vi "Calculator by Eason023.vi"() -> ()   [LabVIEW 2021]
uses:
  <vilib>/regexp/Match Regular Expression.xnode
  <vilib>/gmath/NI_Gmath.lvlib
panel:
  out "Display":string
  in  "C Button":bool
  in  "Stop button":bool
  in  "?":bool
  out "?":bool
  out "?":bool
  out "?":bool
  out "?":bool
  out "?":bool
  out "?":bool
  out "?":bool
  out "?":bool
  out "?":bool
  out "?":bool
  out "?":bool
  out "?":bool
  out "?":bool
  out "?":bool
  out "?":bool
  out "?":bool
  out "?":bool
  out "?":bool
  out "?":bool
  out "?":bool
  out "?":bool
  out "?":bool
  out "?":bool
  out "?":bool
  out "?":bool
  out "?":bool
  out "?":bool
  out "?":bool
  out "?":bool
  out "?":bool
  out "?":bool
  out "?":bool
  out "?":bool
  out "?":bool
  out "?":bool
  out "?":bool
  out "?":bool
  out "?":bool
  out "?":bool
  out "?":bool
  out "?":bool
  out "?":bool
  out "?":bool
  out "?":bool
  out "?":bool
  out "?":bool
  out "?":bool
  out "?":bool
  out "?":bool
  out "?":bool
  out "?":bool
  out "?":bool
  out "?":bool
  out "?":bool
  out "?":bool
  out "?":bool
  out "?":bool
  out "?":bool
  out "?":bool
  out "?":bool
  out "?":bool
  out "?":bool
  out "?":bool
  out "?":bool
  out "?":bool
  out "?":bool
  out "?":bool
  out "?":bool
  out "?":bool
  out "?":bool
  out "?":bool
  out "Elapsed time (s)":u32
  out "Current Time":timestamp
  in  "Load From B Button":bool
  in  "Load From A Button":bool
  in  "Save Button":bool caption="2 Button"
  out "Memory B :":string
  out "Memory A :":string
  in  "1/x Button":bool caption="2 Button"
  in  "≡ Button":bool caption="2 Button"
  in  "+/- Button":bool caption="2 Button"
  in  "CE Button":bool
  in  "\"=\" Button":bool
  out "Syntax Error\nWarning":bool
  in  "Backspace Button":bool
  in  "\")\" Button":bool
  in  "\"(\" Button":bool
  in  "'+' Button":bool caption="2 Button"
  in  "'-' Button":bool caption="2 Button"
  in  "'*' Button":bool caption="2 Button"
  in  "'/' Button":bool caption="2 Button"
  in  "'.' Button":bool caption="2 Button"
  in  "0 Button":bool caption="2 Button"
  in  "8 Button":bool caption="2 Button"
  in  "6 Button":bool caption="2 Button"
  in  "4 Button":bool caption="2 Button"
  in  "9 Button":bool caption="2 Button"
  in  "7 Button":bool caption="2 Button"
  in  "5 Button":bool caption="2 Button"
  in  "3 Button":bool caption="2 Button"
  in  "2 Button":bool
  in  "1 Button":bool
  out "?":bool
  # "七段顯示器 最多10位 (整數與小數各5位) 僅顯示結果 (\"=\"後的數) 超出部分不顯示"
  # "Display mod:\nDetailed----Simple"
  # "Calculator\n          by 113550153"
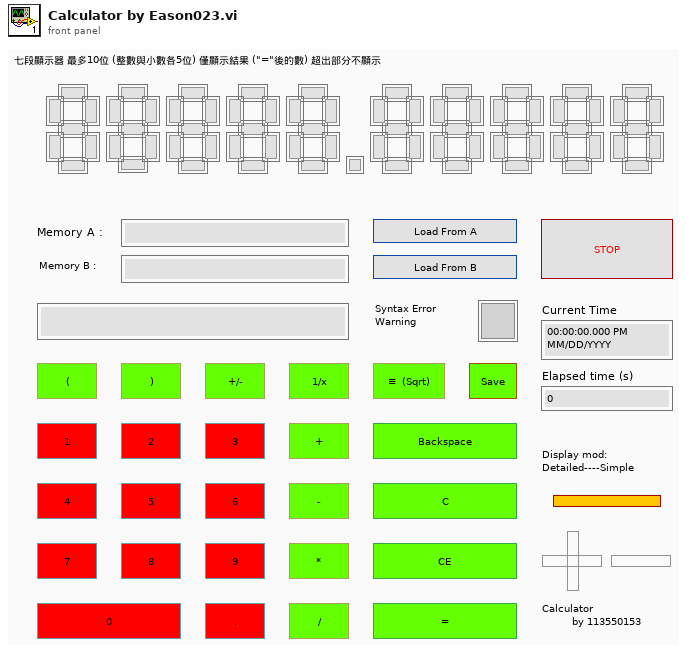
[diagram p1: front panel]
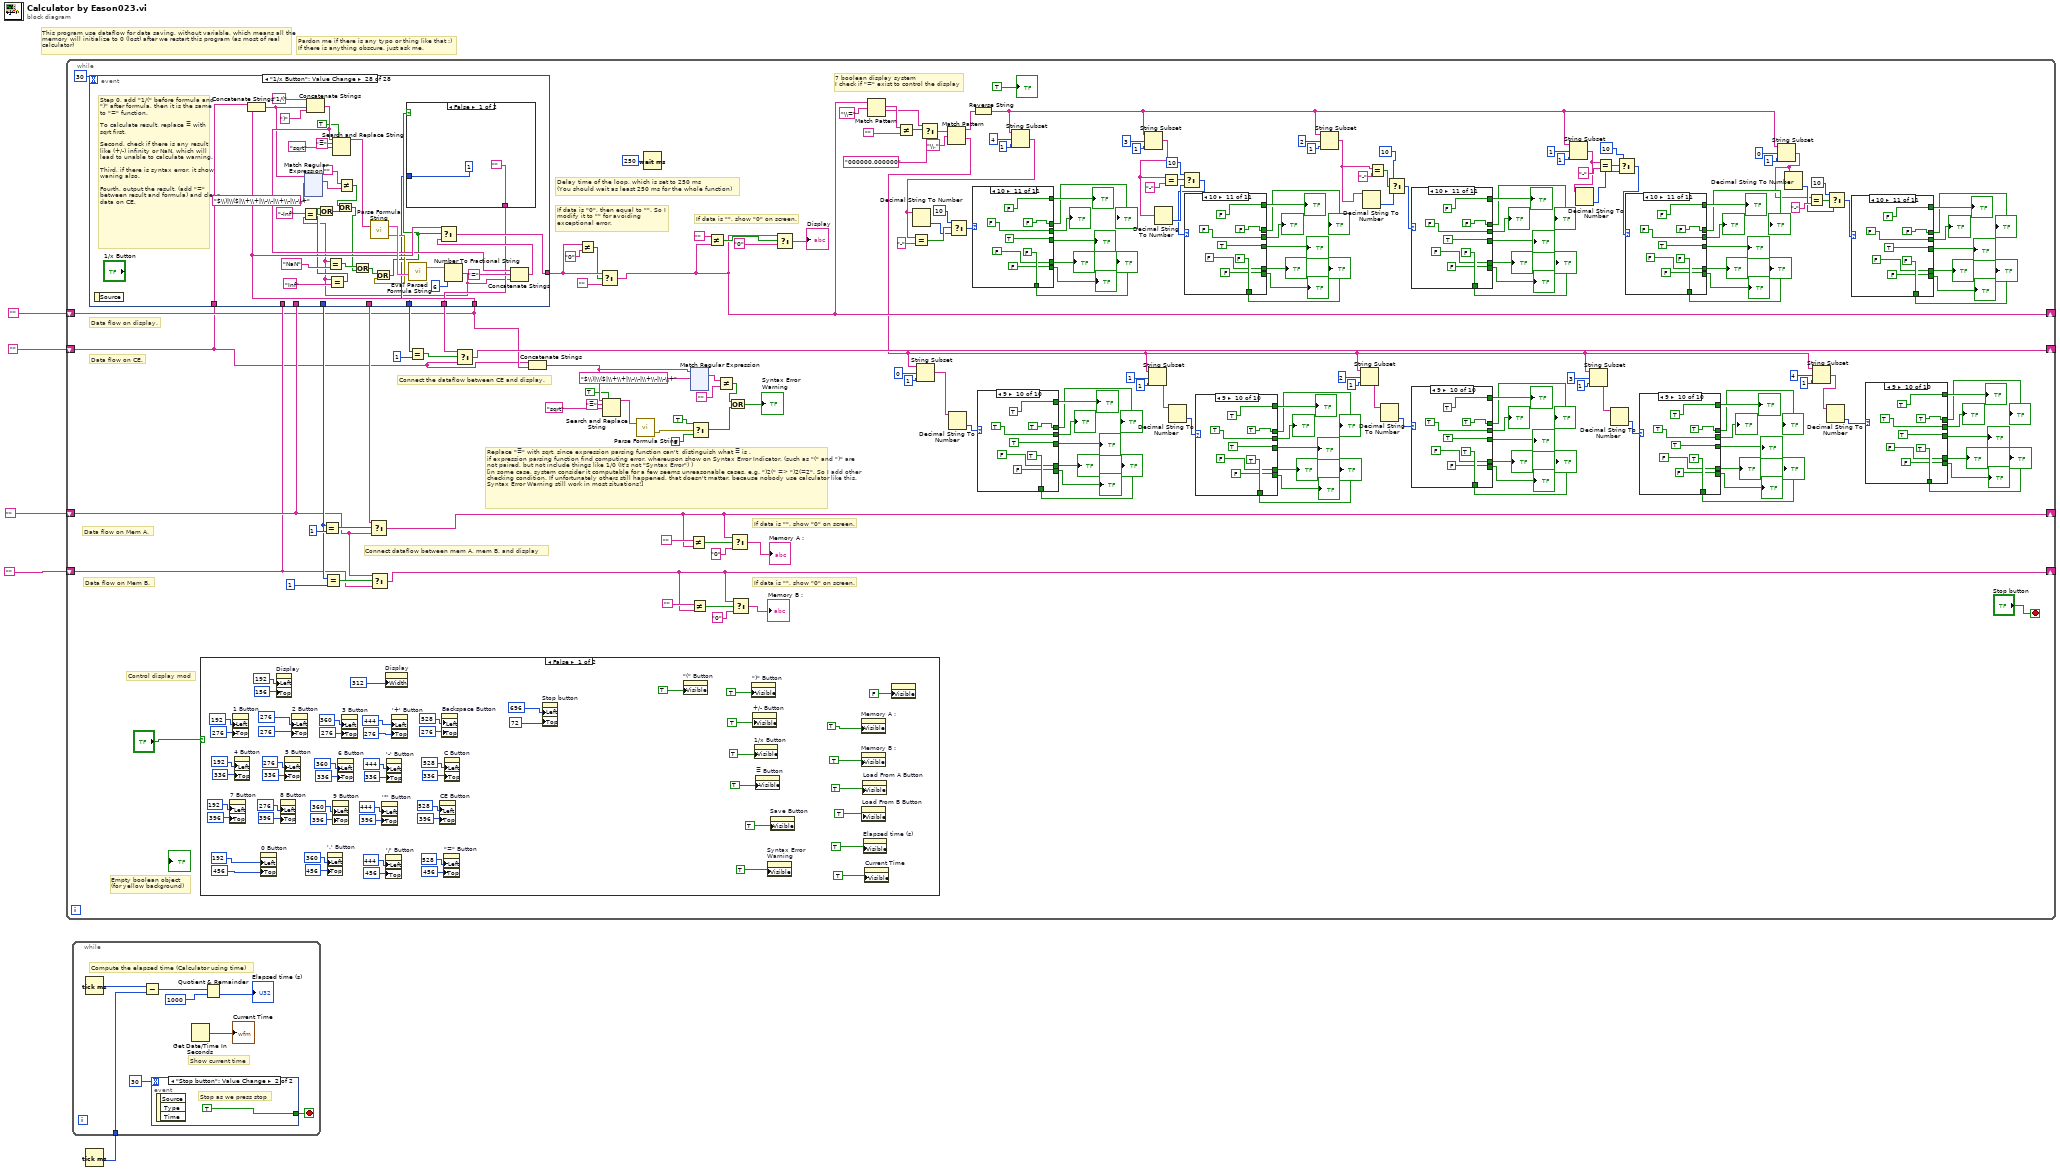
[diagram p0: block diagram]
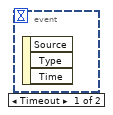
[diagram p2: hidden frame]
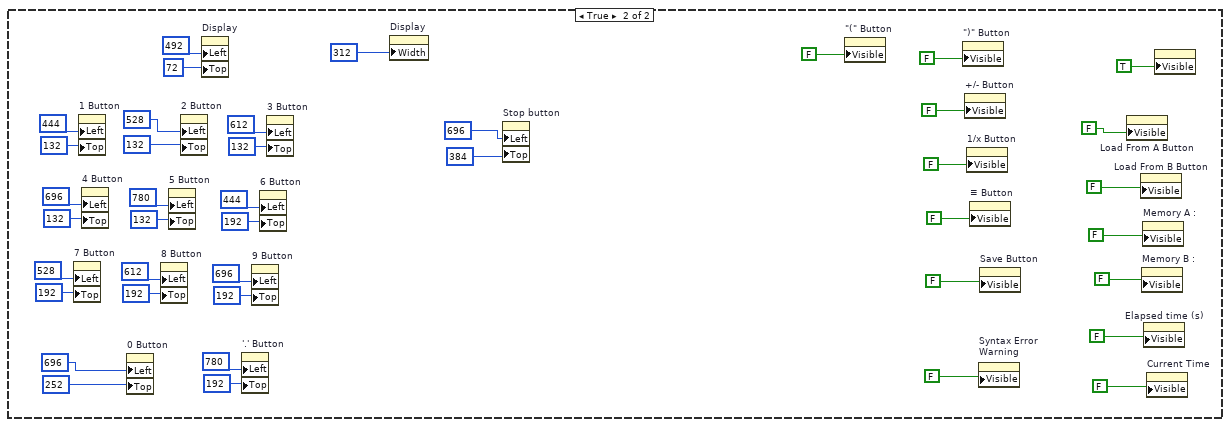
[diagram p3: hidden frame]
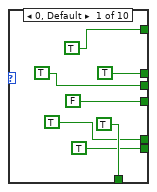
[diagram p4: hidden frame]
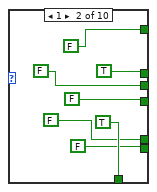
[diagram p5: hidden frame]
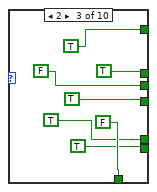
[diagram p6: hidden frame]
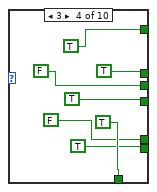
[diagram p7: hidden frame]
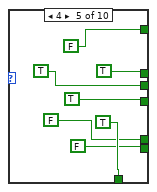
[diagram p8: hidden frame]
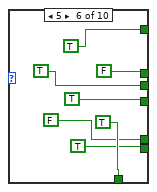
[diagram p9: hidden frame]
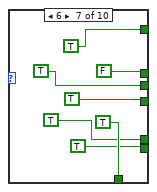
[diagram p10: hidden frame]
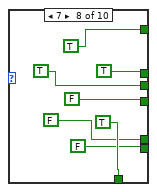
[diagram p11: hidden frame]
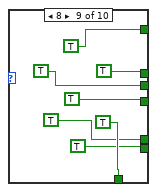
[diagram p12: hidden frame]
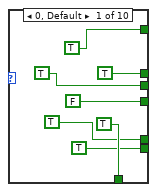
[diagram p13: hidden frame]
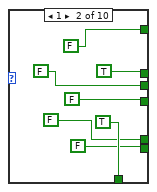
[diagram p14: hidden frame]
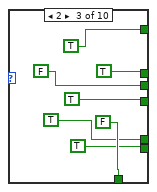
[diagram p15: hidden frame]
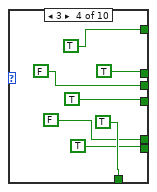
[diagram p16: hidden frame]
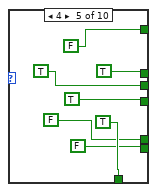
[diagram p17: hidden frame]
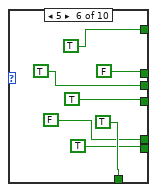
[diagram p18: hidden frame]
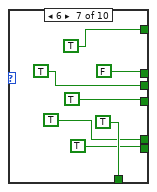
[diagram p19: hidden frame]
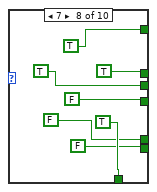
[diagram p20: hidden frame]
diagram:
  # "Pardon me if there is any typo or thing like that :)\nIf there is anything obscure, just ask me."
  # "This program use dataflow for data saving, without variable, which means all the memory will initialize to 0 (lost) after we restart this program (as most of real calculator)"
  n1 = while {
    shift-right: [w156] -> _
    shift-left: "" -> [w161]
    shift-right: [w186] -> _
    shift-left: "" -> [w160]
    shift-right: [w171] -> _
    shift-left: "" -> [w169]
    shift-right: [w173] -> _
    shift-left: "" -> [w168]
    stop <- "Stop button" stop-if-true
    # "Empty boolean object\n(for yellow background)"
    # "Control display mod"
    # "7 boolean display system\nI check if \"=\" exist to control the display"
    # "If data is \"\", show \"0\" on screen."
    # "If data is \"\", show \"0\" on screen."
    # "Connect dataflow between mem A, mem B, and display"
    # "Delay time of the loop, which is set to 250 ms\n(You should wait as least 250 ms for the whole function)"
    # "Connect the dataflow between CE and display."
    # "Replace \"≡\" with sqrt, since expression parsing function can't  distinguish what ≡ is .\nif expression parsing function find computing error, whereupon show on Syntax Error Indicator. (such as \"(\" and \")\" are not paired, but not include things like 1/0 (It's not \"Syntax Error\") )\n[in some case, system consider it computable for a few seems unreasonable cases, e.g. \")2(\" => \")2(=2\". So I add other checking condition. If unfortunately others still happened, that doesn't matter, because nobody use calculator like this. Syntax Error Warning still work in most situations!]"
    # "Data flow on Mem B."
    # "Data flow on Mem A."
    # "Data flow on CE."
    # "Data flow on display."
    # "If data is \"\", show \"0\" on screen."
    # "If data is \"0\", then equal to \"\". So I modify it to \"\" for avoiding\nexceptional error."
    n2 = event shown="[27] \"1/x Button\": Value Change" {
      selector: _ -> [_ _ _ _ _ _ _ _ _ _ _ _ _ _ _ _ _ _ _ _ _ _ _ _ _ _ _ _]
      dyn-events: _ -> [_ _ _ _ _ _ _ _ _ _ _ _ _ _ _ _ _ _ _ _ _ _ _ _ _ _ _ _]
      timeout: 30 -> [_ _ _ _ _ _ _ _ _ _ _ _ _ _ _ _ _ _ _ _ _ _ _ _ _ _ _ _]
      tunnel: w161 -> [w1150 w1152 w1155 w1158 w1161 w1164 w1167 w1170 w1173 w1176 w1179 w1186 w1203 w1206 w1209 w1212 w1215 w1218 w1232 w1354 w1357 w1370 w1372 w1387 _ _ w2040 w2193]
      tunnel: [w1150 w1151 w1154 w1157 w1160 w1163 w1166 w1169 w1172 w1175 w1182 w1196 w1204 w1207 w1210 w1213 w1216 w1219 w1234 "" w1358 w1369 w1372 w1418 w2012 w2013 w2042 w2195] -> w194
      tunnel: [_ _ _ _ _ _ _ _ _ _ _ _ _ _ _ _ _ _ _ i8 1 w1359 _ _ _ _ _ w2029 w2179] -> w189
      tunnel: [_ _ _ _ _ _ _ _ _ _ _ _ _ _ _ _ _ _ _ w1354 w1360 _ _ _ _ _ w2028 w2178] -> w187
      tunnel: [_ _ _ _ _ _ _ _ _ _ _ _ _ _ _ _ _ _ _ _ _ _ i8 1 _ _ _ _ _] -> w181
      tunnel: [_ _ _ _ _ _ _ _ _ _ _ _ _ _ _ _ _ _ _ _ _ _ w1372 _ _ _ _ _] -> w183
      tunnel: w169 -> [_ _ _ _ _ _ _ _ _ _ _ _ _ _ _ _ _ _ _ _ _ _ _ _ w2012 _ _ _]
      tunnel: w168 -> [_ _ _ _ _ _ _ _ _ _ _ _ _ _ _ _ _ _ _ _ _ _ _ _ _ w2013 _ _]
      tunnel: w160 -> [_ _ _ _ _ _ _ _ _ _ _ _ _ _ _ _ _ _ _ _ _ _ _ _ _ _ w2046 w2199]
      event Timeout {
        # "if no button is pressed, then the data flow segue to next section"
        n3 = event-data() -> ()  [unwired: 1 in, 1 out]
      }
      event "1 Button": Value Change {
        # "Add \"1\" to data flow as we press 1 button"
        n4 = event-data() -> ()  [unwired: 1 in, 1 out]
        n5 = Concatenate Strings(w1152, "1") -> (w1151:string)
      }
      event "2 Button": Value Change {
        # "Add \"2\" to data flow as we press 2 button"
        n6 = event-data() -> ()  [unwired: 1 in, 1 out]
        n7 = Concatenate Strings(w1155, "2") -> (w1154:string)
      }
      event "3 Button": Value Change {
        # "Add \"3\" to data flow as we press 3 button"
        n8 = event-data() -> ()  [unwired: 1 in, 1 out]
        n9 = Concatenate Strings(w1158, "3") -> (w1157:string)
      }
      event "4 Button": Value Change {
        # "Add \"4\" to data flow as we press 4 button"
        n10 = event-data() -> ()  [unwired: 1 in, 1 out]
        n11 = Concatenate Strings(w1161, "4") -> (w1160:string)
      }
      event "5 Button": Value Change {
        # "Add \"5\" to data flow as we press 5 button"
        n12 = event-data() -> ()  [unwired: 1 in, 1 out]
        n13 = Concatenate Strings(w1164, "5") -> (w1163:string)
      }
      event "6 Button": Value Change {
        # "Add \"6\" to data flow as we press 6 button"
        n14 = event-data() -> ()  [unwired: 1 in, 1 out]
        n15 = Concatenate Strings(w1167, "6") -> (w1166:string)
      }
      event "7 Button": Value Change {
        # "Add \"7\" to dataflow as we press 7 button"
        n16 = event-data() -> ()  [unwired: 1 in, 1 out]
        n17 = Concatenate Strings(w1170, "7") -> (w1169:string)
      }
      event "8 Button": Value Change {
        # "Add \"8\" to dataflow as we press 8 button"
        n18 = event-data() -> ()  [unwired: 1 in, 1 out]
        n19 = Concatenate Strings(w1173, "8") -> (w1172:string)
      }
      event "9 Button": Value Change {
        # "Add \"9\" to dataflow as we press 9 button"
        n20 = event-data() -> ()  [unwired: 1 in, 1 out]
        n21 = Concatenate Strings(w1176, "9") -> (w1175:string)
      }
      event "0 Button": Value Change {
        # "Add \"0\" to dataflow as we press 0 button.\nIn case we make a \"0\" prefix error, we can't add 0 as there is no data in dataflow"
        n22 = event-data() -> ()  [unwired: 1 in, 1 out]
        n23 = Not Equal?(x="", y=w1179) -> (x != y?=w1180:bool)
        n24 = Concatenate Strings(w1179, "0" ("string")) -> (w1183:string)
        n25 = Select(t=w1183, s=w1180, f="") -> (s? t:f=w1182:string)
      }
      event "'.' Button": Value Change {
        # "Add \".\" to dataflow as we press \".\" button.\nAs there is no data in dataflow we add \".\" and a \"0\" also. (\"0.xxxxxx\")\nAnd a zero before \".\" is mandatory for avoiding exceptional error"
        n26 = event-data() -> ()  [unwired: 1 in, 1 out]
        n27 = String Length(string=w1186) -> (length=w1195:i32)
        n28 = Concatenate Strings(w1186, "0" ("string")) -> (w1187:string)
        n29 = Decrement(x=w1195) -> (x-1=w1194:i32)
        n30 = String Subset(string=w1186, offset (0)=w1194) -> (substring=w1193:string)  [unwired: 1 in]
        n31 = Match Pattern(string=w1193, regular expression="[0-9]+") -> (match substring=w1191:string)  [unwired: 1 in, 3 out]
        n32 = Not Equal?(x="", y=w1186) -> (x != y?=w1199:bool)
        n33 = Not Equal?(x=w1191, y="") -> (x != y?=w1189:bool)
        n34 = Select(t=w1186, s=w1189, f=w1187) -> (s? t:f=w1188:string)
        n35 = Concatenate Strings(w1188, "." ("string")) -> (w1200:string)
        n36 = Select(t=w1200, s=w1199, f="0.") -> (s? t:f=w1196:string)
      }
      event "'+' Button": Value Change {
        # "Add \"+\" to dataflow as we press + button"
        n37 = event-data() -> ()  [unwired: 1 in, 1 out]
        n38 = Concatenate Strings(w1203, "+" ("string")) -> (w1204:string)
      }
      event "'-' Button": Value Change {
        n39 = event-data() -> ()  [unwired: 1 in, 1 out]
        n40 = Concatenate Strings(w1206, "-" ("string")) -> (w1207:string)
      }
      event "'*' Button": Value Change {
        # "Add \"*\" to dataflow as we press * button"
        n41 = event-data() -> ()  [unwired: 1 in, 1 out]
        n42 = Concatenate Strings(w1209, "*" ("string")) -> (w1210:string)
      }
      event "'/' Button": Value Change {
        # "Add \"/\" to dataflow as we press / button"
        n43 = event-data() -> ()  [unwired: 1 in, 1 out]
        n44 = Concatenate Strings(w1212, "/" ("string")) -> (w1213:string)
      }
      event "\"(\" Button": Value Change {
        # "Add \"(\" to dataflow as we press ( button"
        n45 = event-data() -> ()  [unwired: 1 in, 1 out]
        n46 = Concatenate Strings(w1215, "(" ("string")) -> (w1216:string)
      }
      event "\")\" Button": Value Change {
        # "Add \")\" to dataflow as we press ) button"
        n47 = event-data() -> ()  [unwired: 1 in, 1 out]
        n48 = Concatenate Strings(w1218, ")" ("string")) -> (w1219:string)
      }
      event "Backspace Button": Value Change {
        # "Delete the last element as we press Backspace.\nSince length of \"≡\" is 2, so we deal with it by delete 2 character."
        n49 = event-data() -> ()  [unwired: 1 in, 1 out]
        n50 = Not Equal?(x=w1232, y="") -> (x != y?=w1233:bool)
        n51 = Select(t=w1232, s=w1233, f="0") -> (s? t:f=w1221:string)
        n52 = xnode "Match Regular Expression"("input string"=w1221, "regular expression"="≡$") -> ("whole match"=w1222:string)  [unwired: 4 in, 4 out]
        n53 = Not Equal?(x=w1222, y="") -> (x != y?=w1223:bool)
        n54 = String Length(string=w1221) -> (length=w1226:i32)
        n55 = Select(t=2, s=w1223, f=1) -> (s? t:f=w1229:i32)
        n56 = Subtract(x=w1226, y=w1229) -> (x-y=w1225:i32)
        n57 = String Subset(string=w1221, offset (0)=0, length (rest)=w1225) -> (substring=w1230:string)
        n58 = Select(t=w1230, s=w1233, f=w1232) -> (s? t:f=w1234:string)
      }
      event "CE Button": Value Change {
        # "CE function: Move the dataflow from display to CE dataflow, this data will appear as we press \"=\" or \"1/x\" for calculating, but will not appear on display until you calculate result."
        n59 = event-data() -> ()  [unwired: 1 in, 1 out]
      }
      event "C Button": Value Change {
        # "Check before delete data, if \"yes\" then drop current data (include CE dataflow) and create new empty data, otherwise not."
        n60 = event-data() -> ()  [unwired: 1 in, 1 out]
        n61 = Two Button Dialog(message="Are you sure to clear?", 1:"No" ("F button name (\"Cancel\")"), 2:"Yes" ("T button name (\"OK\")")) -> (T button?=w1361:bool)
        n62 = case shown="True" w1361 {
          tunnel: [_ ""] -> w1360
          tunnel: [_ i8 1] -> w1359
          tunnel: [w1365 ""] -> w1358
          tunnel: w1357 -> [w1365 _]
          frame False {
          }
          frame True {
          }
        }
      }
      event "≡ Button": Value Change {
        # "Add ≡( as we press ≡ button"
        n63 = event-data() -> ()  [unwired: 1 in, 1 out]
        n64 = Concatenate Strings(w1370, "≡(" ("string")) -> (w1369:string)
      }
      event "Save Button": Value Change {
        # "Duplicate display dataflow to mem dataflow"
        n65 = event-data() -> ()  [unwired: 1 in, 1 out]
      }
      event "+/- Button": Value Change {
        # "Since it is somewhat complicate, I am going to illustrate the main idea only (or you can ask me also) ; )\nThis part, I try to match ( ) as last element is \")\", if it is possible to find (-x.x) or (-x), then change it to positive.\nIf it is x.x or x, change it to negative. x is a number here."
        n66 = event-data() -> ()  [unwired: 1 in, 1 out]
        n67 = Reverse String(1:w1387) -> (0:w1415:string)
        n68 = String Length(string=w1387) -> (length=w1426:i32)
        n69 = Decrement(x=w1426) -> (x-1=w1425:i32)
        n70 = xnode "Match Regular Expression"("input string"=w1415, "regular expression"="[0-9]+") -> ("whole match"=w1404:string, "after match"=w1397:string)  [unwired: 4 in, 3 out]
        n71 = String Subset(string=w1387, offset (0)=w1425) -> (substring=w1416:string)  [unwired: 1 in]
        n72 = Reverse String(1:w1387) -> (0:w1395:string)
        n73 = String Subset(string=w1397, length (rest)=1 ("length (rest)")) -> (substring=w1409:string)  [unwired: 1 in]
        n74 = Equal?(x=w1409, y=".") -> (x = y?=w1400:bool)
        n75 = xnode "Match Regular Expression"("input string"=w1395, "regular expression"="\\)[0-9]+\\.[0-9]+\\-\\(|\\)[0-9]+\\-\\(") -> ("whole match"=w1385:string)  [unwired: 4 in, 4 out]
        n76 = xnode "Match Regular Expression"("input string"=w1415, "regular expression"="\\)[0-9]+\\.[0-9]+\\-\\(|\\)[0-9]+\\-\\(") -> ("whole match"=w1377:string, "after match"=w1382:string)  [unwired: 4 in, 3 out]
        n77 = xnode "Match Regular Expression"("input string"=w1397, "regular expression"="\\.[0-9]+") -> ("whole match"=w1406:string, "after match"=w1399:string)  [unwired: 4 in, 3 out]
        n78 = Select(t=w1406, s=w1400, f="") -> (s? t:f=w1403:string)
        n79 = Concatenate Strings(w1404, w1403) -> (w1401:string)
        n80 = String Length(string=w1387) -> (length=w1392:i32)
        n81 = String Length(string=w1385) -> (length=w1394:i32)
        n82 = String Length(string=w1377) -> (length=w1375:i32)
        n83 = Subtract(x=w1392, y=w1394) -> (x-y=w1393:i32)
        n84 = Reverse String(1:w1385) -> (0:w1386:string)
        n85 = Subtract(x=w1375, y=3) -> (x-y=w1376:i32)
        n86 = Select(t=w1399, s=w1400, f=w1397) -> (s? t:f=w1398:string)
        n87 = String Subset(string=w1387, offset (0)=w1393) -> (substring=w1390:string)  [unwired: 1 in]
        n88 = String Subset(string=w1377, offset (0)=1, length (rest)=w1376) -> (substring=w1378:string)
        n89 = xnode "Match Regular Expression"("input string"=w1416, "regular expression"="[0-9]+") -> ("whole match"=w1422:string)  [unwired: 4 in, 4 out]
        n90 = Not Equal?(x=w1390, y="") -> (x != y?=w1388:bool)
        n91 = Equal?(x=w1386, y=w1390) -> (x = y?=w1389:bool)
        n92 = Concatenate Strings(w1378, w1382) -> (w1381:string)
        n93 = Concatenate Strings(")" ("string"), w1401, "-(" ("string"), w1398) -> (w1402:string)
        n94 = And(x=w1389, y=w1388) -> (x .and. y?=w1391:bool)
        n95 = Reverse String(1:w1381) -> (0:w1380:string)
        n96 = Reverse String(1:w1402) -> (0:w1414:string)
        n97 = Not(x=w1391) -> (.not. x?=w1419:bool)
        n98 = Equal?(x=w1422, y="") -> (x = y?=w1420:bool)
        n99 = Select(t=w1380, s=w1391, f=w1414) -> (s? t:f=w1417:string)
        n100 = And(x=w1420, y=w1419) -> (x .and. y?=w1421:bool)
        n101 = Select(t=w1387, s=w1421, f=w1417) -> (s? t:f=w1418:string)
      }
      event "Load From A Button": Value Change {
        # "Make display data flow being the data in mem A."
        n102 = event-data() -> ()  [unwired: 1 in, 1 out]
      }
      event "Load From B Button": Value Change {
        # "Make display data flow being the data in mem B."
        n103 = event-data() -> ()  [unwired: 1 in, 1 out]
      }
      event "\"=\" Button": Value Change {
        w2015 = ""
        # "To calculate result, replace ≡ with sqrt first.\n \nSecond, check if there is any result like (+/-) infinity or NaN, which will lead to unable to calculate warning. \n\nThird, if there is syntax error, it show waning also.\n\nFourth, output the result, (add \"=\" between result and formula) and clear data on CE."
        n104 = event-data() -> ()  [unwired: 1 in, 1 out]
        n105 = Concatenate Strings(w2046, w2040) -> (w2016:string)
        n106 = xnode "Match Regular Expression"("input string"=w2016, "regular expression"="$\\)|\\($|\\+\\+|\\-\\-|\\+\\-|\\-\\+") -> ("whole match"=w2020:string)  [unwired: 4 in, 4 out]
        n107 = Not Equal?(x=w2020, y=w2015) -> (x != y?=w2021:bool)
        n108 = Equal?(x=w2016, y=w2015) -> (x = y?=w2017:bool)
        n109 = Search and Replace String(replace all?=TRUE ("replace all? (F)"), input string=w2016, search string="≡", replace string="sqrt" ("replace string (\"\")")) -> (result string=w2036:string)  [unwired: 4 in, 3 out]
        n110 = call <vilib>:"Parse Formula String.vi"("formula"=w2036) -> ("error out"=w2031:errorcluster, "Parsed Formula"=w2041:cluster{"Table":i32[][], "Y Values":dbl[]})  [unwired: 1 in]
        n111 = call <vilib>:"Eval Parsed Formula String.vi"("Parsed Formula"=w2041) -> ("y value"=w2045:dbl)  [unwired: 3 in, 1 out]
        n112 = Number To Fractional String(number=w2045, precision (6)=i16 6) -> (F-format string=w2025:string)  [unwired: 2 in]
        n113 = Equal?(x=w2025, y="-Inf") -> (x = y?=w2026:bool)
        n114 = Equal?(x=w2025, y="NaN") -> (x = y?=w2034:bool)
        n115 = Equal?(x=w2025, y="Inf") -> (x = y?=w2024:bool)
        n116 = Or(x=w2024, y=w2026) -> (x .or. y?=w2023:bool)
        n117 = Or(x=w2021, y=w2023) -> (x .or. y?=w2019:bool)
        n118 = Or(x=w2017, y=w2019) -> (x .or. y?=w2018:bool)
        n119 = Or(x=w2034, y=w2018) -> (x .or. y?=w2035:bool)
        n120 = Or(x=w2035, y=w2031) -> (x .or. y?=w2030:bool)
        n121 = case shown="False" w2030 {
          tunnel: [i8 1 _] -> w2029
          tunnel: ["" _] -> w2028
          frame False {
          }
          frame True {
            n122 = call "Display Message to User"() -> ()  [unwired: 10 in, 2 out]
          }
        }
        n123 = Concatenate Strings(w2016, "=" ("string"), w2025) -> (w2038:string)
        n124 = Select(t=w2040, s=w2030, f=w2038) -> (s? t:f=w2042:string)
      }
      event "1/x Button": Value Change {
        # "Step 0, add \"1/(\" before formula and \")\" after formula, then it is the same to \"=\" function.\n\nTo calculate result, replace ≡ with sqrt first.\n \nSecond, check if there is any result like (+/-) infinity or NaN, which will lead to unable to calculate warning. \n\nThird, if there is syntax error, it show waning also.\n\nFourth, output the result, (add \"=\" between result and formula) and clear data on CE."
        n125 = event-data() -> ()  [unwired: 1 in, 1 out]
        n126 = Concatenate Strings(w2199, w2193) -> (w2172:string)
        n127 = xnode "Match Regular Expression"("input string"=w2172, "regular expression"="$\\)|\\($|\\+\\+|\\-\\-|\\+\\-|\\-\\+") -> ("whole match"=w2169:string)  [unwired: 4 in, 4 out]
        n128 = Concatenate Strings("1/(" ("string"), w2172, ")" ("string")) -> (w2186:string)
        n129 = Search and Replace String(replace all?=TRUE ("replace all? (F)"), input string=w2186, search string="≡", replace string="sqrt" ("replace string (\"\")")) -> (result string=w2187:string)  [unwired: 4 in, 3 out]
        n130 = Not Equal?(x="", y=w2169) -> (x != y?=w2167:bool)
        n131 = call <vilib>:"Parse Formula String.vi"("formula"=w2187) -> ("error out"=w2181:errorcluster, "Parsed Formula"=w2194:cluster{"Table":i32[][], "Y Values":dbl[]})  [unwired: 1 in]
        n132 = call <vilib>:"Eval Parsed Formula String.vi"("Parsed Formula"=w2194) -> ("y value"=w2198:dbl)  [unwired: 3 in, 1 out]
        n133 = Number To Fractional String(number=w2198, precision (6)=i16 6) -> (F-format string=w2175:string)  [unwired: 2 in]
        n134 = Equal?(x="-Inf", y=w2175) -> (x = y?=w2177:bool)
        n135 = Equal?(x=w2175, y="NaN") -> (x = y?=w2185:bool)
        n136 = Equal?(x=w2175, y="Inf") -> (x = y?=w2176:bool)
        n137 = Or(x=w2176, y=w2177) -> (x .or. y?=w2171:bool)
        n138 = Or(x=w2167, y=w2171) -> (x .or. y?=w2170:bool)
        n139 = Or(x=w2185, y=w2170) -> (x .or. y?=w2184:bool)
        n140 = Or(x=w2184, y=w2181) -> (x .or. y?=w2180:bool)
        n141 = case shown="False" w2180 {
          tunnel: [i8 1 _] -> w2179
          tunnel: ["" _] -> w2178
          frame False {
          }
          frame True {
            n142 = call "Display Message to User2"() -> ()  [unwired: 10 in, 2 out]
          }
        }
        n143 = Concatenate Strings(w2186, "=" ("string"), w2175) -> (w2191:string)
        n144 = Select(t=w2193, s=w2180, f=w2191) -> (s? t:f=w2195:string)
      }
    }
    n145 = case shown="False" "?" {
      frame False {
        n146 = property on="7 Button" class="Bool"("Left"=192, "Top"=396) -> ()  [unwired: 2 in, 2 out]
        n147 = property on="1 Button" class="Bool"("Left"=192, "Top"=276) -> ()  [unwired: 2 in, 2 out]
        n148 = property on="4 Button" class="Bool"("Left"=192, "Top"=336) -> ()  [unwired: 2 in, 2 out]
        n149 = property on="0 Button" class="Bool"("Left"=192, "Top"=456) -> ()  [unwired: 2 in, 2 out]
        n150 = property on="Display" class="Str"("Left"=192, "Top"=156) -> ()  [unwired: 2 in, 2 out]
        n151 = property on="8 Button" class="Bool"("Left"=276, "Top"=396) -> ()  [unwired: 2 in, 2 out]
        n152 = property on="5 Button" class="Bool"("Left"=276, "Top"=336) -> ()  [unwired: 2 in, 2 out]
        n153 = property on="2 Button" class="Bool"("Left"=276, "Top"=276) -> ()  [unwired: 2 in, 2 out]
        n154 = property on="'.' Button" class="Bool"("Left"=360, "Top"=456) -> ()  [unwired: 2 in, 2 out]
        n155 = property on="9 Button" class="Bool"("Left"=360, "Top"=396) -> ()  [unwired: 2 in, 2 out]
        n156 = property on="6 Button" class="Bool"("Left"=360, "Top"=336) -> ()  [unwired: 2 in, 2 out]
        n157 = property on="3 Button" class="Bool"("Left"=360, "Top"=276) -> ()  [unwired: 2 in, 2 out]
        n158 = property on="'*' Button" class="Bool"("Left"=444, "Top"=396) -> ()  [unwired: 2 in, 2 out]
        n159 = property on="Display" class="Str"("Width"=u32 312) -> ()  [unwired: 2 in, 2 out]
        n160 = property on="'/' Button" class="Bool"("Left"=444, "Top"=456) -> ()  [unwired: 2 in, 2 out]
        n161 = property on="'-' Button" class="Bool"("Left"=444, "Top"=336) -> ()  [unwired: 2 in, 2 out]
        n162 = property on="'+' Button" class="Bool"("Left"=444, "Top"=276) -> ()  [unwired: 2 in, 2 out]
        n163 = property on="CE Button" class="Bool"("Left"=528, "Top"=396) -> ()  [unwired: 2 in, 2 out]
        n164 = property on="Backspace Button" class="Bool"("Left"=528, "Top"=276) -> ()  [unwired: 2 in, 2 out]
        n165 = property on="\"=\" Button" class="Bool"("Left"=528, "Top"=456) -> ()  [unwired: 2 in, 2 out]
        n166 = property on="C Button" class="Bool"("Left"=528, "Top"=336) -> ()  [unwired: 2 in, 2 out]
        n167 = property on="Stop button" class="Bool"("Left"=696, "Top"=72) -> ()  [unwired: 2 in, 2 out]
        n168 = property on="\"(\" Button" class="Bool"("Visible"=TRUE) -> ()  [unwired: 2 in, 2 out]
        n169 = property on="\")\" Button" class="Bool"("Visible"=TRUE) -> ()  [unwired: 2 in, 2 out]
        n170 = property on="+/- Button" class="Bool"("Visible"=TRUE) -> ()  [unwired: 2 in, 2 out]
        n171 = property on="1/x Button" class="Bool"("Visible"=TRUE) -> ()  [unwired: 2 in, 2 out]
        n172 = property on="≡ Button" class="Bool"("Visible"=TRUE) -> ()  [unwired: 2 in, 2 out]
        n173 = property on="Syntax Error\nWarning" class="Bool (strict)"("Visible"=TRUE) -> ()  [unwired: 2 in, 2 out]
        n174 = property on="Save Button" class="Bool"("Visible"=TRUE) -> ()  [unwired: 2 in, 2 out]
        n175 = property on="Memory A :" class="Str"("Visible"=TRUE) -> ()  [unwired: 2 in, 2 out]
        n176 = property on="Memory B :" class="Str"("Visible"=TRUE) -> ()  [unwired: 2 in, 2 out]
        n177 = property on="Load From B Button" class="Bool"("Visible"=TRUE) -> ()  [unwired: 2 in, 2 out]
        n178 = property on="Load From A Button" class="Bool"("Visible"=TRUE) -> ()  [unwired: 2 in, 2 out]
        n179 = property on="Elapsed time (s)" class="DigNum (strict)"("Visible"=TRUE) -> ()  [unwired: 2 in, 2 out]
        n180 = property on="Current Time" class="AbsTime (strict)"("Visible"=TRUE) -> ()  [unwired: 2 in, 2 out]
        n181 = property class="Bool (strict)"("Visible"=FALSE) -> ()  [unwired: 2 in, 2 out]
      }
      frame True {
        n182 = property on="7 Button" class="Bool"("Left"=528, "Top"=192) -> ()  [unwired: 2 in, 2 out]
        n183 = property on="1 Button" class="Bool"("Left"=444, "Top"=132) -> ()  [unwired: 2 in, 2 out]
        n184 = property on="4 Button" class="Bool"("Left"=696, "Top"=132) -> ()  [unwired: 2 in, 2 out]
        n185 = property on="0 Button" class="Bool"("Left"=696, "Top"=252) -> ()  [unwired: 2 in, 2 out]
        n186 = property on="8 Button" class="Bool"("Left"=612, "Top"=192) -> ()  [unwired: 2 in, 2 out]
        n187 = property on="5 Button" class="Bool"("Left"=780, "Top"=132) -> ()  [unwired: 2 in, 2 out]
        n188 = property on="2 Button" class="Bool"("Left"=528, "Top"=132) -> ()  [unwired: 2 in, 2 out]
        n189 = property on="Display" class="Str"("Left"=492, "Top"=72) -> ()  [unwired: 2 in, 2 out]
        n190 = property on="'.' Button" class="Bool"("Left"=780, "Top"=192) -> ()  [unwired: 2 in, 2 out]
        n191 = property on="9 Button" class="Bool"("Left"=696, "Top"=192) -> ()  [unwired: 2 in, 2 out]
        n192 = property on="6 Button" class="Bool"("Left"=444, "Top"=192) -> ()  [unwired: 2 in, 2 out]
        n193 = property on="3 Button" class="Bool"("Left"=612, "Top"=132) -> ()  [unwired: 2 in, 2 out]
        n194 = property on="Display" class="Str"("Width"=u32 312) -> ()  [unwired: 2 in, 2 out]
        n195 = property on="Stop button" class="Bool"("Left"=696, "Top"=384) -> ()  [unwired: 2 in, 2 out]
        n196 = property on="\"(\" Button" class="Bool"("Visible"=FALSE) -> ()  [unwired: 2 in, 2 out]
        n197 = property on="\")\" Button" class="Bool"("Visible"=FALSE) -> ()  [unwired: 2 in, 2 out]
        n198 = property on="+/- Button" class="Bool"("Visible"=FALSE) -> ()  [unwired: 2 in, 2 out]
        n199 = property on="1/x Button" class="Bool"("Visible"=FALSE) -> ()  [unwired: 2 in, 2 out]
        n200 = property on="≡ Button" class="Bool"("Visible"=FALSE) -> ()  [unwired: 2 in, 2 out]
        n201 = property on="Syntax Error\nWarning" class="Bool (strict)"("Visible"=FALSE) -> ()  [unwired: 2 in, 2 out]
        n202 = property on="Save Button" class="Bool"("Visible"=FALSE) -> ()  [unwired: 2 in, 2 out]
        n203 = property on="Load From A Button" class="Bool"("Visible"=FALSE) -> ()  [unwired: 2 in, 2 out]
        n204 = property on="Load From B Button" class="Bool"("Visible"=FALSE) -> ()  [unwired: 2 in, 2 out]
        n205 = property on="Memory B :" class="Str"("Visible"=FALSE) -> ()  [unwired: 2 in, 2 out]
        n206 = property on="Memory A :" class="Str"("Visible"=FALSE) -> ()  [unwired: 2 in, 2 out]
        n207 = property on="Elapsed time (s)" class="DigNum (strict)"("Visible"=FALSE) -> ()  [unwired: 2 in, 2 out]
        n208 = property on="Current Time" class="AbsTime (strict)"("Visible"=FALSE) -> ()  [unwired: 2 in, 2 out]
        n209 = property class="Bool (strict)"("Visible"=TRUE) -> ()  [unwired: 2 in, 2 out]
      }
    }
    n210 = Equal?(x=w181, y=i8 1) -> (x = y?=w184:bool)
    n211 = Equal?(x=w181, y=i8 1) -> (x = y?=w180:bool)
    n212 = Select(t=w183, s=w184, f=w169) -> (s? t:f=w171:string)
    n213 = Select(t=w169, s=w180, f=w168) -> (s? t:f=w173:string)
    n214 = Equal?(x=w189, y=i8 1) -> (x = y?=w188:bool)
    n215 = Select(t=w187, s=w188, f=w160) -> (s? t:f=w186:string)
    n216 = Concatenate Strings(w160, w161) -> (w38:string)
    n217 = Not Equal?(x=w194, y="0") -> (x != y?=w192:bool)
    n218 = Select(t=w194, s=w192, f="") -> (s? t:f=w156:string)
    n219 = Search and Replace String(replace all?=TRUE ("replace all? (F)"), input string=w38, search string="≡", replace string="sqrt" ("replace string (\"\")")) -> (result string=w165:string)  [unwired: 4 in, 3 out]
    n220 = call <vilib>:"Parse Formula String.vi"("formula"=w165) -> ("error out"=w162:errorcluster)  [unwired: 1 in, 1 out]
    n221 = Wait (ms)(milliseconds to wait=u32 250) -> ()  [unwired: 1 out]
    n222 = Not Equal?(x="", y=w171) -> (x != y?=w175:bool)
    n223 = xnode "Match Regular Expression"("input string"=w38, "regular expression"="$\\)|\\($|\\+\\+|\\-\\-|\\+\\-|\\-\\+") -> ("whole match"=w40:string)  [unwired: 4 in, 4 out]
    n224 = Not Equal?(x="", y=w173) -> (x != y?=w178:bool)
    n225 = Select(t=TRUE, s=w162, f=FALSE) -> (s? t:f=w43:bool)
    n226 = Not Equal?(x="", y=w156) -> (x != y?=w195:bool)
    n227 = Not Equal?(x=w40, y="") -> (x != y?=w41:bool)
    n228 = Or(x=w41, y=w43) -> (x .or. y?=→"Syntax Error\nWarning":bool)
    n229 = Select(t=w171, s=w175, f="0") -> (s? t:f=→"Memory A :":string)
    n230 = Select(t=w173, s=w178, f="0") -> (s? t:f=→"Memory B :":string)
    n231 = Select(t=w156, s=w195, f="0") -> (s? t:f=→"Display":string)
    n232 = Match Pattern(string=w156, regular expression="\\=") -> (match substring=w154:string, after substring=w152:string)  [unwired: 1 in, 2 out]
    n233 = Not Equal?(x=w154, y="") -> (x != y?=w157:bool)
    n234 = Select(t=w152, s=w157, f="000000.000000") -> (s? t:f=w150:string)
    n235 = Match Pattern(string=w150, regular expression="\\.") -> (before substring=w131:string, after substring=w132:string)  [unwired: 1 in, 2 out]
    n236 = String Subset(string=w132, offset (0)=0, length (rest)=1 ("length (rest)")) -> (substring=w137:string)
    n237 = Decimal String To Number(string=w137) -> (number=w77:i32)  [unwired: 2 in, 1 out]
    n238 = Reverse String(1:w131) -> (0:w120:string)
    n239 = case shown="9" w77 {
      tunnel: [TRUE FALSE TRUE TRUE FALSE TRUE TRUE TRUE TRUE TRUE] -> w84
      tunnel: [TRUE TRUE TRUE TRUE TRUE FALSE FALSE TRUE TRUE TRUE] -> w83
      tunnel: [FALSE FALSE TRUE TRUE TRUE TRUE TRUE FALSE TRUE TRUE] -> w82
      tunnel: [TRUE TRUE FALSE TRUE TRUE TRUE TRUE TRUE TRUE TRUE] -> w81
      tunnel: [TRUE FALSE TRUE TRUE FALSE TRUE TRUE FALSE TRUE FALSE] -> w80
      tunnel: [TRUE FALSE TRUE FALSE FALSE FALSE TRUE FALSE TRUE FALSE] -> w79
      tunnel: [TRUE FALSE FALSE FALSE TRUE TRUE TRUE TRUE TRUE TRUE] -> w78
      frame 0, Default {
      }
      frame 1 {
      }
      frame 2 {
      }
      frame 3 {
      }
      frame 4 {
      }
      frame 5 {
      }
      frame 6 {
      }
      frame 7 {
      }
      frame 8 {
      }
      frame 9 {
      }
    }
    "?" <- w84
    "?" <- w82
    "?" <- w80
    "?" <- w83
    "?" <- w79
    "?" <- w81
    "?" <- w78
    n240 = String Subset(string=w120, offset (0)=4, length (rest)=1 ("length (rest)")) -> (substring=w36:string)
    n241 = Decimal String To Number(string=w36) -> (number=w33:i32)  [unwired: 2 in, 1 out]
    n242 = Equal?(x=w36, y="-") -> (x = y?=w34:bool)
    n243 = Select(t=10, s=w34, f=w33) -> (s? t:f=w31:i32)
    n244 = case shown="10" w31 {
      tunnel: [TRUE FALSE TRUE TRUE FALSE TRUE TRUE TRUE TRUE TRUE FALSE] -> w119
      tunnel: [TRUE TRUE TRUE TRUE TRUE FALSE FALSE TRUE TRUE TRUE FALSE] -> w118
      tunnel: [FALSE FALSE TRUE TRUE TRUE TRUE TRUE FALSE TRUE TRUE TRUE] -> w117
      tunnel: [TRUE TRUE FALSE TRUE TRUE TRUE TRUE TRUE TRUE TRUE FALSE] -> w116
      tunnel: [TRUE FALSE TRUE TRUE FALSE TRUE TRUE FALSE TRUE FALSE FALSE] -> w115
      tunnel: [TRUE FALSE TRUE FALSE FALSE FALSE TRUE FALSE TRUE FALSE FALSE] -> w114
      tunnel: [TRUE FALSE FALSE FALSE TRUE TRUE TRUE TRUE TRUE TRUE FALSE] -> w113
      frame 0, Default {
      }
      frame 1 {
      }
      frame 2 {
      }
      frame 3 {
      }
      frame 4 {
      }
      frame 5 {
      }
      frame 6 {
      }
      frame 7 {
      }
      frame 8 {
      }
      frame 9 {
      }
      frame 10 {
      }
    }
    "?" <- w119
    "?" <- w117
    "?" <- w115
    "?" <- w118
    "?" <- w114
    "?" <- w116
    "?" <- w113
    n245 = String Subset(string=w120, offset (0)=3, length (rest)=1 ("length (rest)")) -> (substring=w27:string)
    n246 = String Subset(string=w132, offset (0)=1, length (rest)=1 ("length (rest)")) -> (substring=w136:string)
    n247 = Decimal String To Number(string=w27) -> (number=w26:i32)  [unwired: 2 in, 1 out]
    n248 = Equal?(x=w27, y="-") -> (x = y?=w28:bool)
    n249 = Decimal String To Number(string=w136) -> (number=w69:i32)  [unwired: 2 in, 1 out]
    n250 = Select(t=10, s=w28, f=w26) -> (s? t:f=w25:i32)
    n251 = case shown="10" w25 {
      tunnel: [TRUE FALSE TRUE TRUE FALSE TRUE TRUE TRUE TRUE TRUE FALSE] -> w112
      tunnel: [TRUE TRUE TRUE TRUE TRUE FALSE FALSE TRUE TRUE TRUE FALSE] -> w111
      tunnel: [FALSE FALSE TRUE TRUE TRUE TRUE TRUE FALSE TRUE TRUE TRUE] -> w110
      tunnel: [TRUE TRUE FALSE TRUE TRUE TRUE TRUE TRUE TRUE TRUE FALSE] -> w109
      tunnel: [TRUE FALSE TRUE TRUE FALSE TRUE TRUE FALSE TRUE FALSE FALSE] -> w108
      tunnel: [TRUE FALSE TRUE FALSE FALSE FALSE TRUE FALSE TRUE FALSE FALSE] -> w107
      tunnel: [TRUE FALSE FALSE FALSE TRUE TRUE TRUE TRUE TRUE TRUE FALSE] -> w106
      frame 0, Default {
      }
      frame 1 {
      }
      frame 2 {
      }
      frame 3 {
      }
      frame 4 {
      }
      frame 5 {
      }
      frame 6 {
      }
      frame 7 {
      }
      frame 8 {
      }
      frame 9 {
      }
      frame 10 {
      }
    }
    "?" <- w112
    "?" <- w110
    "?" <- w108
    "?" <- w111
    "?" <- w107
    "?" <- w109
    "?" <- w106
    n252 = case shown="9" w69 {
      tunnel: [TRUE FALSE TRUE TRUE FALSE TRUE TRUE TRUE TRUE TRUE] -> w76
      tunnel: [TRUE TRUE TRUE TRUE TRUE FALSE FALSE TRUE TRUE TRUE] -> w75
      tunnel: [FALSE FALSE TRUE TRUE TRUE TRUE TRUE FALSE TRUE TRUE] -> w74
      tunnel: [TRUE TRUE FALSE TRUE TRUE TRUE TRUE TRUE TRUE TRUE] -> w73
      tunnel: [TRUE FALSE TRUE TRUE FALSE TRUE TRUE FALSE TRUE FALSE] -> w72
      tunnel: [TRUE FALSE TRUE FALSE FALSE FALSE TRUE FALSE TRUE FALSE] -> w71
      tunnel: [TRUE FALSE FALSE FALSE TRUE TRUE TRUE TRUE TRUE TRUE] -> w70
      frame 0, Default {
      }
      frame 1 {
      }
      frame 2 {
      }
      frame 3 {
      }
      frame 4 {
      }
      frame 5 {
      }
      frame 6 {
      }
      frame 7 {
      }
      frame 8 {
      }
      frame 9 {
      }
    }
    "?" <- w76
    "?" <- w74
    "?" <- w72
    "?" <- w75
    "?" <- w71
    "?" <- w73
    "?" <- w70
    n253 = String Subset(string=w120, offset (0)=2, length (rest)=1 ("length (rest)")) -> (substring=w21:string)
    n254 = String Subset(string=w132, offset (0)=2, length (rest)=1 ("length (rest)")) -> (substring=w135:string)
    n255 = Decimal String To Number(string=w21) -> (number=w20:i32)  [unwired: 2 in, 1 out]
    n256 = Equal?(x=w21, y="-") -> (x = y?=w22:bool)
    n257 = Decimal String To Number(string=w135) -> (number=w61:i32)  [unwired: 2 in, 1 out]
    n258 = Select(t=10, s=w22, f=w20) -> (s? t:f=w19:i32)
    n259 = case shown="10" w19 {
      tunnel: [TRUE FALSE TRUE TRUE FALSE TRUE TRUE TRUE TRUE TRUE FALSE] -> w105
      tunnel: [TRUE TRUE TRUE TRUE TRUE FALSE FALSE TRUE TRUE TRUE FALSE] -> w104
      tunnel: [FALSE FALSE TRUE TRUE TRUE TRUE TRUE FALSE TRUE TRUE TRUE] -> w103
      tunnel: [TRUE TRUE FALSE TRUE TRUE TRUE TRUE TRUE TRUE TRUE FALSE] -> w102
      tunnel: [TRUE FALSE TRUE TRUE FALSE TRUE TRUE FALSE TRUE FALSE FALSE] -> w101
      tunnel: [TRUE FALSE TRUE FALSE FALSE FALSE TRUE FALSE TRUE FALSE FALSE] -> w100
      tunnel: [TRUE FALSE FALSE FALSE TRUE TRUE TRUE TRUE TRUE TRUE FALSE] -> w99
      frame 0, Default {
      }
      frame 1 {
      }
      frame 2 {
      }
      frame 3 {
      }
      frame 4 {
      }
      frame 5 {
      }
      frame 6 {
      }
      frame 7 {
      }
      frame 8 {
      }
      frame 9 {
      }
      frame 10 {
      }
    }
    "?" <- w105
    "?" <- w103
    "?" <- w101
    "?" <- w104
    "?" <- w100
    "?" <- w102
    "?" <- w99
    n260 = case shown="9" w61 {
      tunnel: [TRUE FALSE TRUE TRUE FALSE TRUE TRUE TRUE TRUE TRUE] -> w68
      tunnel: [TRUE TRUE TRUE TRUE TRUE FALSE FALSE TRUE TRUE TRUE] -> w67
      tunnel: [FALSE FALSE TRUE TRUE TRUE TRUE TRUE FALSE TRUE TRUE] -> w66
      tunnel: [TRUE TRUE FALSE TRUE TRUE TRUE TRUE TRUE TRUE TRUE] -> w65
      tunnel: [TRUE FALSE TRUE TRUE FALSE TRUE TRUE FALSE TRUE FALSE] -> w64
      tunnel: [TRUE FALSE TRUE FALSE FALSE FALSE TRUE FALSE TRUE FALSE] -> w63
      tunnel: [TRUE FALSE FALSE FALSE TRUE TRUE TRUE TRUE TRUE TRUE] -> w62
      frame 0, Default {
      }
      frame 1 {
      }
      frame 2 {
      }
      frame 3 {
      }
      frame 4 {
      }
      frame 5 {
      }
      frame 6 {
      }
      frame 7 {
      }
      frame 8 {
      }
      frame 9 {
      }
    }
    "?" <- w68
    "?" <- w66
    "?" <- w64
    "?" <- w67
    "?" <- w63
    "?" <- w65
    "?" <- w62
    n261 = String Subset(string=w120, offset (0)=1, length (rest)=1 ("length (rest)")) -> (substring=w14:string)
    n262 = Decimal String To Number(string=w14) -> (number=w15:i32)  [unwired: 2 in, 1 out]
    n263 = String Subset(string=w132, offset (0)=3, length (rest)=1 ("length (rest)")) -> (substring=w134:string)
    n264 = Equal?(x=w14, y="-") -> (x = y?=w16:bool)
    n265 = Decimal String To Number(string=w134) -> (number=w53:i32)  [unwired: 2 in, 1 out]
    n266 = Select(t=10, s=w16, f=w15) -> (s? t:f=w13:i32)
    n267 = case shown="10" w13 {
      tunnel: [TRUE FALSE TRUE TRUE FALSE TRUE TRUE TRUE TRUE TRUE FALSE] -> w98
      tunnel: [TRUE TRUE TRUE TRUE TRUE FALSE FALSE TRUE TRUE TRUE FALSE] -> w97
      tunnel: [FALSE FALSE TRUE TRUE TRUE TRUE TRUE FALSE TRUE TRUE TRUE] -> w96
      tunnel: [TRUE TRUE FALSE TRUE TRUE TRUE TRUE TRUE TRUE TRUE FALSE] -> w95
      tunnel: [TRUE FALSE TRUE TRUE FALSE TRUE TRUE FALSE TRUE FALSE FALSE] -> w94
      tunnel: [TRUE FALSE TRUE FALSE FALSE FALSE TRUE FALSE TRUE FALSE FALSE] -> w93
      tunnel: [TRUE FALSE FALSE FALSE TRUE TRUE TRUE TRUE TRUE TRUE FALSE] -> w92
      frame 0, Default {
      }
      frame 1 {
      }
      frame 2 {
      }
      frame 3 {
      }
      frame 4 {
      }
      frame 5 {
      }
      frame 6 {
      }
      frame 7 {
      }
      frame 8 {
      }
      frame 9 {
      }
      frame 10 {
      }
    }
    "?" <- w98
    "?" <- w96
    "?" <- w94
    "?" <- w97
    "?" <- w93
    "?" <- w95
    "?" <- w92
    n268 = case shown="9" w53 {
      tunnel: [TRUE FALSE TRUE TRUE FALSE TRUE TRUE TRUE TRUE TRUE] -> w60
      tunnel: [TRUE TRUE TRUE TRUE TRUE FALSE FALSE TRUE TRUE TRUE] -> w59
      tunnel: [FALSE FALSE TRUE TRUE TRUE TRUE TRUE FALSE TRUE TRUE] -> w58
      tunnel: [TRUE TRUE FALSE TRUE TRUE TRUE TRUE TRUE TRUE TRUE] -> w57
      tunnel: [TRUE FALSE TRUE TRUE FALSE TRUE TRUE FALSE TRUE FALSE] -> w56
      tunnel: [TRUE FALSE TRUE FALSE FALSE FALSE TRUE FALSE TRUE FALSE] -> w55
      tunnel: [TRUE FALSE FALSE FALSE TRUE TRUE TRUE TRUE TRUE TRUE] -> w54
      frame 0, Default {
      }
      frame 1 {
      }
      frame 2 {
      }
      frame 3 {
      }
      frame 4 {
      }
      frame 5 {
      }
      frame 6 {
      }
      frame 7 {
      }
      frame 8 {
      }
      frame 9 {
      }
    }
    "?" <- w60
    "?" <- w58
    "?" <- w56
    "?" <- w59
    "?" <- w55
    "?" <- w57
    "?" <- w54
    n269 = String Subset(string=w120, offset (0)=0, length (rest)=1 ("length (rest)")) -> (substring=w8:string)
    n270 = Decimal String To Number(string=w8) -> (number=w9:i32)  [unwired: 2 in, 1 out]
    n271 = Equal?(x=w8, y="-") -> (x = y?=w10:bool)
    n272 = String Subset(string=w132, offset (0)=4, length (rest)=1 ("length (rest)")) -> (substring=w133:string)
    n273 = Decimal String To Number(string=w133) -> (number=w45:i32)  [unwired: 2 in, 1 out]
    n274 = Select(t=10, s=w10, f=w9) -> (s? t:f=w7:i32)
    n275 = case shown="10" w7 {
      tunnel: [TRUE FALSE TRUE TRUE FALSE TRUE TRUE TRUE TRUE TRUE FALSE] -> w91
      tunnel: [TRUE TRUE TRUE TRUE TRUE FALSE FALSE TRUE TRUE TRUE FALSE] -> w90
      tunnel: [FALSE FALSE TRUE TRUE TRUE TRUE TRUE FALSE TRUE TRUE TRUE] -> w89
      tunnel: [TRUE TRUE FALSE TRUE TRUE TRUE TRUE TRUE TRUE TRUE FALSE] -> w88
      tunnel: [TRUE FALSE TRUE TRUE FALSE TRUE TRUE FALSE TRUE FALSE FALSE] -> w87
      tunnel: [TRUE FALSE TRUE FALSE FALSE FALSE TRUE FALSE TRUE FALSE FALSE] -> w86
      tunnel: [TRUE FALSE FALSE FALSE TRUE TRUE TRUE TRUE TRUE TRUE FALSE] -> w85
      frame 0, Default {
      }
      frame 1 {
      }
      frame 2 {
      }
      frame 3 {
      }
      frame 4 {
      }
      frame 5 {
      }
      frame 6 {
      }
      frame 7 {
      }
      frame 8 {
      }
      frame 9 {
      }
      frame 10 {
      }
    }
    "?" <- w91
    "?" <- w89
    "?" <- w87
    "?" <- w90
    "?" <- w86
    "?" <- w88
    "?" <- w85
    n276 = case shown="9" w45 {
      tunnel: [TRUE FALSE TRUE TRUE FALSE TRUE TRUE TRUE TRUE TRUE] -> w52
      tunnel: [TRUE TRUE TRUE TRUE TRUE FALSE FALSE TRUE TRUE TRUE] -> w51
      tunnel: [FALSE FALSE TRUE TRUE TRUE TRUE TRUE FALSE TRUE TRUE] -> w50
      tunnel: [TRUE TRUE FALSE TRUE TRUE TRUE TRUE TRUE TRUE TRUE] -> w49
      tunnel: [TRUE FALSE TRUE TRUE FALSE TRUE TRUE FALSE TRUE FALSE] -> w48
      tunnel: [TRUE FALSE TRUE FALSE FALSE FALSE TRUE FALSE TRUE FALSE] -> w47
      tunnel: [TRUE FALSE FALSE FALSE TRUE TRUE TRUE TRUE TRUE TRUE] -> w46
      frame 0, Default {
      }
      frame 1 {
      }
      frame 2 {
      }
      frame 3 {
      }
      frame 4 {
      }
      frame 5 {
      }
      frame 6 {
      }
      frame 7 {
      }
      frame 8 {
      }
      frame 9 {
      }
    }
    "?" <- w52
    "?" <- w50
    "?" <- w48
    "?" <- w51
    "?" <- w47
    "?" <- w49
    "?" <- w46
    "?" <- TRUE
  }
  n277 = Tick Count (ms)() -> (millisecond timer value=w1:u32)
  n278 = while {
    tunnel: w1 -> [w2321]
    stop <- w2320 stop-if-true
    # "Compute the elapsed time (Calculator using time)"
    # "Show current time"
    n279 = Tick Count (ms)() -> (millisecond timer value=w2325:u32)
    n280 = Subtract(x=w2325, y=w2321) -> (x-y=w2323:u32)
    n281 = event shown="[1] \"Stop button\": Value Change" {
      selector: _ -> [_ _]
      dyn-events: _ -> [_ _]
      timeout: 30 -> [_ _]
      tunnel: [_ TRUE] -> w2320
      event Timeout {
        n282 = event-data() -> ()  [unwired: 1 in, 3 out]
      }
      event "Stop button": Value Change {
        # "Stop as we press stop"
        n283 = event-data() -> ()  [unwired: 1 in, 3 out]
      }
    }
    n284 = Get Date/Time In Seconds() -> (seconds since 1Jan1904=→"Current Time":timestamp)
    n285 = Quotient & Remainder(x=w2323, y=u32 1000) -> (floor(x/y)=→"Elapsed time (s)":u32)  [unwired: 1 out]
  }
